vi "Create_Object.vi"(8 "error in (no error)":errorcluster, 9 "Block Diagram in":T1, 10 "owner refnum":variant, 11 "For Loop in":refnum<class "For Loop.lvclass">) -> (0 "error out":errorcluster, 1 "Block Diagram Out":T1, 3 "For Loop out":refnum<class "For Loop.lvclass">)   [LabVIEW 2025, in "For Loop.lvclass"]
uses:
  For Loop.lvclass
  C:/Users/mrjak/Documents/GitHub/LVGPT/LabVIEW/VIs/Classes/Node/Node.lvclass
  Controls/bd.ctl
  Node.lvclass
  Controls/wire.ctl
  Controls/Terminal.ctl
  Node.lvclass/Node.ctl
  Loop.lvclass
  For Loop.lvclass/For Loop.ctl
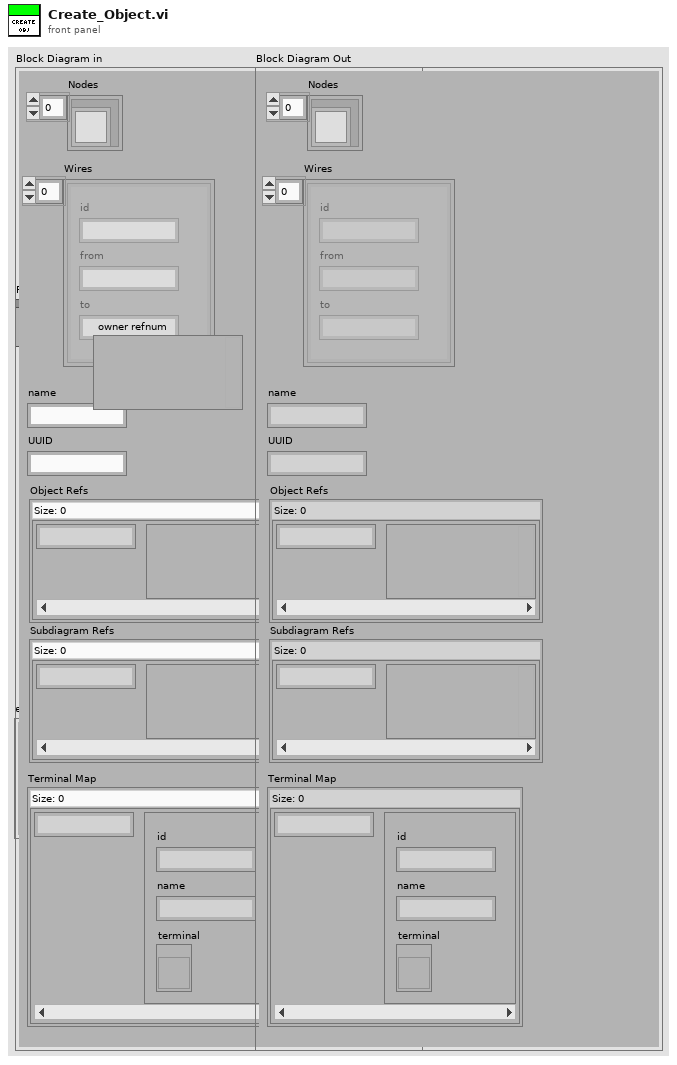
[diagram p1: front panel]
types:
  T1 = typedef "bd.ctl" = cluster{"Nodes":refnum<class "Node.lvclass">[], "Wires":T2[], "name":string, "UUID":string, "Object Refs":map{string, variant}, "Subdiagram Refs":map{string, variant}, "Terminal Map":map{string, T3}}
  T2 = typedef "wire.ctl" = cluster{"id":string, "from":string, "to":string}
  T3 = typedef "Terminal.ctl" = cluster{"id":string, "name":string, "terminal":refnum<vi>}
  T4 = typedef "Subdiagram.ctl" = cluster{"diagram":refnum<vi>, "selector":string, "uuid":string}
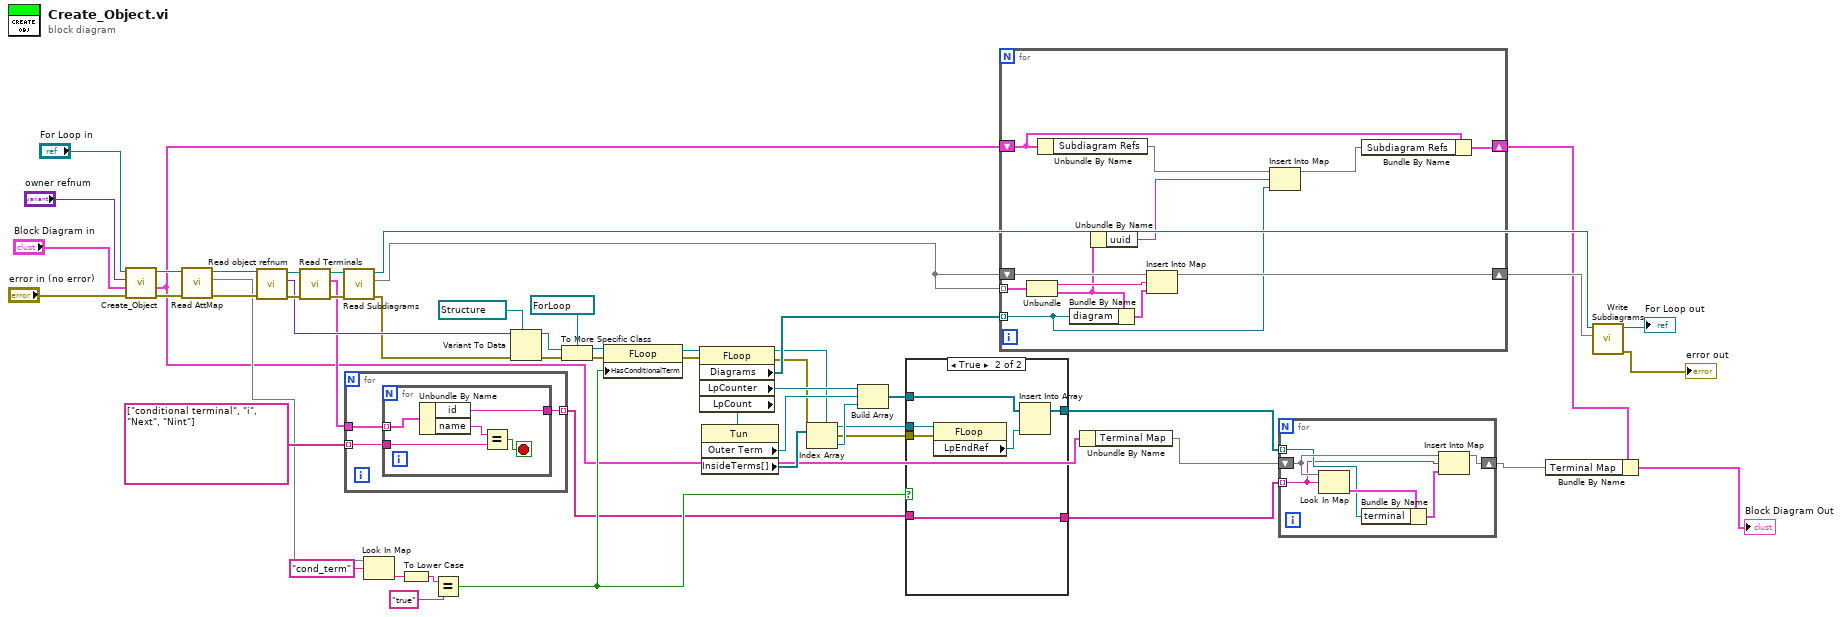
[diagram p0: block diagram]
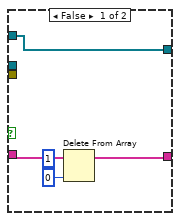
[diagram p2: hidden frame]
diagram:
  n1 = call-parent "Create_Object.vi"("error in (no error)"="error in (no error)", "Block Diagram in"="Block Diagram in", "owner refnum"="owner refnum", "Loop in"="For Loop in") -> ("error out"=w24:errorcluster, "Block Diagram Out"=w3:T1, "Loop out"=w31:refnum<class "For Loop.lvclass">)  [unwired: 5 in]
  n2 = call "Read AttMap.vi"("error in (no error)"=w24, "Node in"=w31) -> ("error out"=w23:errorcluster, "AttMap"=w22:map{string, string}, "Node out"=w25:refnum<class "For Loop.lvclass">)  [unwired: 7 in]
  n3 = call-dynamic "Read object refnum.vi"("error in (no error)"=w23, "Node in"=w25) -> ("error out"=w47:errorcluster, "object refnum"=w41:variant, "Node out"=w48:refnum<class "For Loop.lvclass">)  [unwired: 7 in]
  n4 = call "Read Terminals.vi"("error in (no error)"=w47, "Node in"=w48) -> ("error out"=w42:errorcluster, "Terminals"=w35:T3[], "Node out"=w45:refnum<class "For Loop.lvclass">)  [unwired: 7 in]
  n5 = call-dynamic "Read Subdiagrams.vi"("error in (no error)"=w42, "Structure in"=w45) -> ("error out"=w40:errorcluster, "Subdiagrams"=w44:map{string, T4}, "Structure out"=w43:refnum<class "For Loop.lvclass">)  [unwired: 7 in]
  n6 = for {
    tunnel: w35 -> [w55]
    tunnel: [w54] -> w7 mode=indexing
    tunnel: string[] ["conditional terminal", "i", "Next", "Nint"] -> [w53] mode=indexing
    n7 = for {
      tunnel: w55 -> [w60] mode=indexing
      tunnel: [w58] -> w54
      tunnel: w53 -> [w57]
      stop <- w56 stop-if-true
      n8 = Unbundle By Name(w60) -> ("id"=w58:string, "name"=w59:string)
      n9 = Equal?(x=w59, y=w57) -> (x = y?=w56:bool)
    }
  }
  n10 = Look In Map(map=w22, key="cond_term") -> (value=w20:string)  [unwired: 1 in, 1 out]
  n11 = To Lower Case(string=w20) -> (all lower case string=w19:string)
  n12 = Equal?(x=w19, y="true") -> (x = y?=w15:bool)
  n13 = Variant To Data(error in=w40, type=refnum<vi> refnum ("vi object class"), Variant=w41) -> (data=w36:refnum<vi>, error out=w39:errorcluster)
  n14 = To More Specific Class(target class=refnum<vi> refnum ("vi object class"), reference=w36, error in=w39) -> (specific class reference=w16:refnum<vi>, error out=w17:errorcluster)
  n15 = property class="FLoop"(reference=w16, error in=w17, "HasConditionalTerm"=w15) -> (reference out=w13:refnum<vi>, error out=w14:errorcluster)
  n16 = property class="FLoop"(reference=w13, error in=w14) -> (reference out=w10:refnum<vi>, error out=w11:errorcluster, "Diagrams"=w12:refnum<vi>[], "LpCounter"=w34:refnum<vi>, "LpCount"=w29:refnum<vi>)
  n17 = property class="Tun"(reference=w29) -> ("Outer Term"=w28:refnum<vi>, "InsideTerms[]"=w27:refnum<vi>[])  [unwired: 1 in, 2 out]
  n18 = Index Array(array=w27) -> (element=w26:refnum<vi>)  [unwired: 1 in]
  n19 = Build Array(w34, w28, w26) -> (w9:refnum<vi>[])
  n20 = case shown="True" w15 {
    tunnel: w11 -> [_ w70]
    tunnel: w10 -> [_ w71]
    tunnel: w9 -> [w65 w69]
    tunnel: [w65 w67] -> w8
    tunnel: w7 -> [w64 w66]
    tunnel: [w61 w66] -> w6
    frame False {
      n21 = Delete From Array(array=w64, length=1, index=0) -> (array with subset deleted=w61:string[])  [unwired: 1 out]
    }
    frame True {
      n22 = property class="FLoop"(reference=w71, error in=w70) -> ("LpEndRef"=w68:refnum<vi>)  [unwired: 2 out]
      n23 = Insert Into Array(array=w69, new element=w68) -> (w67:refnum<vi>[])  [unwired: 1 in]
    }
  }
  n24 = for {
    tunnel: w12 -> [w72] mode=indexing
    tunnel: w44 -> [w83] mode=indexing
    shift-right: [w79] -> w46
    shift-left: w44 -> [w82]
    shift-right: [w77] -> w2
    shift-left: w3 -> [w78]
    n25 = Unbundle(w83) -> ("String"=w80:string, "Subdiagram"=w74:T4)
    n26 = Unbundle By Name(w78) -> ("Subdiagram Refs"=w76:map{string, variant})
    n27 = Bundle By Name(cluster=w74, "diagram"=w72) -> (w81:T4)
    n28 = Unbundle By Name(w74) -> ("uuid"=w73:string)
    n29 = Insert Into Map(map in=w82, key=w80, value=w81) -> (map out=w79:map{string, T4})  [unwired: 2 out]
    n30 = Insert Into Map(map in=w76, key=w73, value=w72) -> (map out=w75:map{string, variant})  [unwired: 2 out]
    n31 = Bundle By Name(cluster=w78, "Subdiagram Refs"=w75) -> (w77:T1)
  }
  n32 = Unbundle By Name(w3) -> ("Terminal Map"=w5:map{string, T3})
  n33 = for {
    tunnel: w8 -> [w87] mode=indexing
    tunnel: w6 -> [w84] mode=indexing
    shift-right: [w85] -> w1
    shift-left: w5 -> [w89]
    n34 = Look In Map(map=w89, key=w84) -> (value=w88:T3)  [unwired: 1 in, 1 out]
    n35 = Bundle By Name(cluster=w88, "terminal"=w87) -> (w86:T3)
    n36 = Insert Into Map(map in=w89, key=w84, value=w86) -> (map out=w85:map{string, T3})  [unwired: 2 out]
  }
  n37 = Bundle By Name(cluster=w2, "Terminal Map"=w1) -> (→"Block Diagram Out":T1)
  n38 = call-dynamic "Write Subdiagrams.vi"("Subdiagrams"=w46, "Structure in"=w43) -> ("error out"=→"error out":errorcluster, "Structure out"=→"For Loop out":refnum<class "For Loop.lvclass">)  [unwired: 8 in]
